vi "Configure Serial Bus (I2S - Basic).vi"(0 "VISA resource name":refnum<visa-resource-name>, 1 "Receiver Data Width (4 bits)":dbl=4.0, 2 "WS Polarity (0: Left)":i32(ring) items=["Left", "Right"], 5 "Serial Bus Name (1: Serial Bus 1)":i32(ring)=1 items=["Serial Bus 1"=1, "Serial Bus 2"=2], 7 "Display Base (0: Decimal)":i32(ring) items=["Decimal", "Hex"], 9 "Clock Edge (0: Negative)":i32(ring) items=["Negative", "Positive"], 11 "error in (no error)":errorcluster, 12 "Transmitted Data Width (4 bits)":dbl=4.0, 13 "Data Alignment (0: I2S)":i32(ring) items=["I2S", "Left Justified", "Right Justified"]) -> (4 "VISA resource name out":refnum<visa-resource-name>, 15 "error out":errorcluster)   [LabVIEW 2015, in "Agilent 2000 3000 X-Series.lvlib"]
doc: "Configures the basic settings of I2S bus.\n\nNote:\nThis VI is not supported by 1000 X-Series"
uses:
  Agilent 2000 3000 X-Series.lvlib
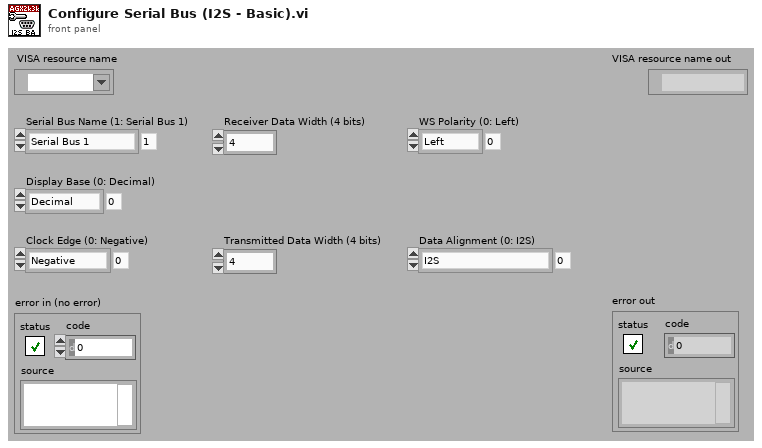
[diagram p1: front panel]
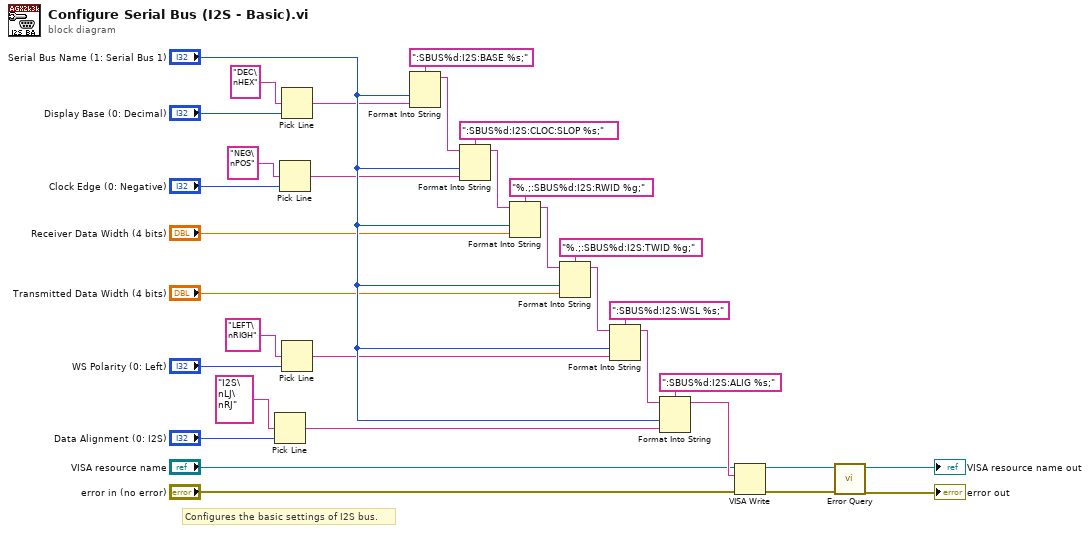
[diagram p0: block diagram]
diagram:
  # "Configures the basic settings of I2S bus."
  n1 = Pick Line(multi-line string="I2S\nLJ\nRJ", line index="Data Alignment (0: I2S)") -> (output string=w8:string)  [unwired: 1 out]
  n2 = Pick Line(multi-line string="NEG\nPOS", line index="Clock Edge (0: Negative)") -> (output string=w24:string)  [unwired: 1 out]
  n3 = Pick Line(multi-line string="DEC\nHEX", line index="Display Base (0: Decimal)") -> (output string=w29:string)  [unwired: 1 out]
  n4 = Pick Line(multi-line string="LEFT\nRIGH", line index="WS Polarity (0: Left)") -> (output string=w13:string)  [unwired: 1 out]
  n5 = Format Into String(format string=":SBUS%d:I2S:BASE %s;", "Serial Bus Name (1: Serial Bus 1)", w29) -> (resulting string=w26:string)  [unwired: 2 in, 1 out]
  n6 = Format Into String(format string=":SBUS%d:I2S:CLOC:SLOP %s;", initial string=w26, "Serial Bus Name (1: Serial Bus 1)", w24) -> (resulting string=w23:string)  [unwired: 1 in, 1 out]
  n7 = Format Into String(format string="%.;:SBUS%d:I2S:RWID %g;", initial string=w23, "Serial Bus Name (1: Serial Bus 1)", "Receiver Data Width (4 bits)") -> (resulting string=w20:string)  [unwired: 1 in, 1 out]
  n8 = Format Into String(format string="%.;:SBUS%d:I2S:TWID %g;", initial string=w20, "Serial Bus Name (1: Serial Bus 1)", "Transmitted Data Width (4 bits)") -> (resulting string=w15:string)  [unwired: 1 in, 1 out]
  n9 = Format Into String(format string=":SBUS%d:I2S:WSL %s;", initial string=w15, "Serial Bus Name (1: Serial Bus 1)", w13) -> (resulting string=w10:string)  [unwired: 1 in, 1 out]
  n10 = Format Into String(format string=":SBUS%d:I2S:ALIG %s;", initial string=w10, "Serial Bus Name (1: Serial Bus 1)", w8) -> (resulting string=w7:string)  [unwired: 1 in, 1 out]
  n11 = VISA Write(VISA resource name="VISA resource name", write buffer=w7, error in (no error)="error in (no error)") -> (VISA resource name out=w4:refnum<visa-resource-name>, error out=w3:errorcluster)  [unwired: 1 out]
  n12 = call "Error Query.vi"("error in (no error)"=w3, "VISA resource name"=w4) -> ("error out"=→"error out":errorcluster, "VISA resource name out"=→"VISA resource name out":refnum<visa-resource-name>)  [unwired: 8 out]
